vi "Run.vi"(8 "error in (no error)":errorcluster caption="entrée d'erreur (pas d'erreur)", 9 "labels":string[][](array[string]), 10 "X":string[][](array[string]), 11 "Davies_Bouldin_Score.lvclass":refnum<class "Davies_Bouldin_Score.lvclass">) -> (0 "error out":errorcluster caption="sortie d'erreur", 2 "Score":string, 3 "Davies_Bouldin_Score.lvclass":refnum<class "Davies_Bouldin_Score.lvclass">)   [LabVIEW 2020, in "Davies_Bouldin_Score.lvclass"]
doc: "Returns :\n\n- score : float\nThe resulting Davies-Bouldin score."
uses:
  Davies_Bouldin_Score.lvclass
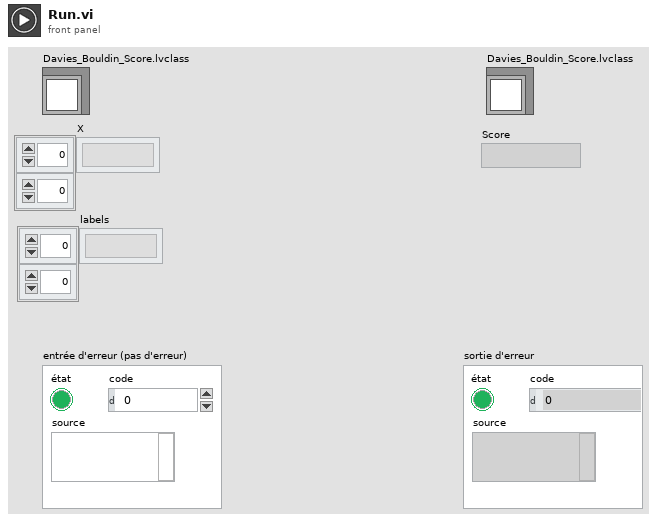
[diagram p1: front panel]
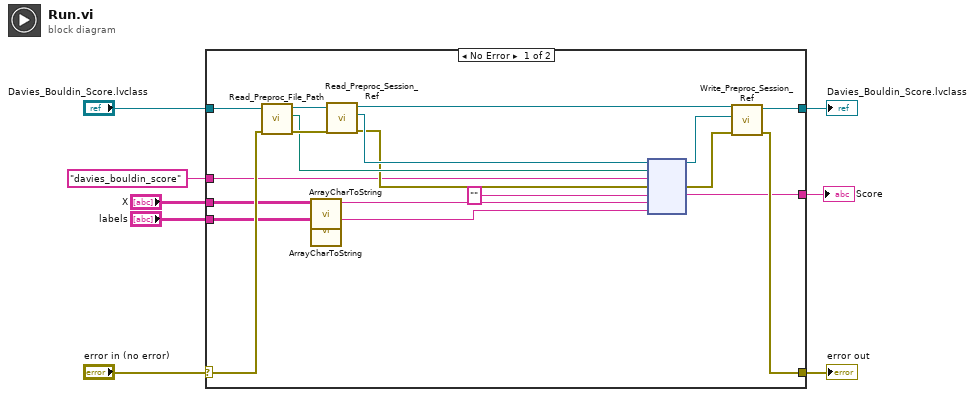
[diagram p0: block diagram]
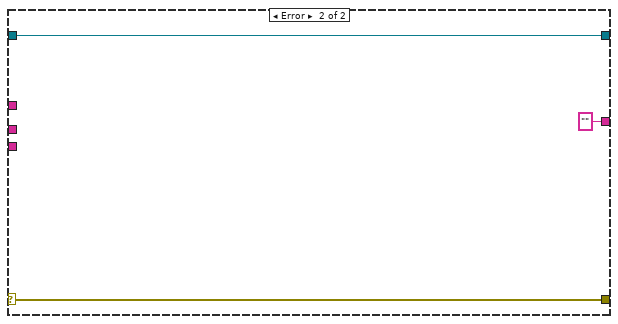
[diagram p2: hidden frame]
diagram:
  n1 = case shown="No Error" "error in (no error)" {
    selector: "error in (no error)" -> [w16 w30]
    tunnel: [w17 w30] -> w7
    tunnel: [w18 w29] -> w5
    tunnel: "Davies_Bouldin_Score.lvclass" -> [w13 w29]
    tunnel: "davies_bouldin_score" -> [w15 _]
    tunnel: [w14 ""] -> w4
    tunnel: "X" -> [w12 _]
    tunnel: "labels" -> [w11 _]
    frame No Error {
      n2 = call-dynamic "Read_Preproc_File_Path.vi"("error in (no error)"=w16, "Python in"=w13) -> ("error out"=w26:errorcluster, "File_Path"=w25:path, "Python out"=w27:refnum<class "Davies_Bouldin_Score.lvclass">)  [unwired: 7 in]
      n3 = call "ArrayCharToString.vi"("TAB"=w12) -> ("Instruction"=w10:string)  [unwired: 10 in]
      n4 = call "ArrayCharToString.vi"("TAB"=w11) -> ("Instruction"=w9:string)  [unwired: 10 in]
      n5 = call-dynamic "Read_Preproc_Session_Ref.vi"("error in (no error)"=w26, "Python in"=w27) -> ("error out"=w23:errorcluster, "Session_ref"=w24:refnum<k35>, "Python out"=w22:refnum<class "Davies_Bouldin_Score.lvclass">)  [unwired: 7 in]
      n6 = node(w24, w25, w15, w23, "", w10, w9) -> (w20:refnum<k35>, w21:errorcluster, w14:string)  [unwired: 2 in, 2 out]
      n7 = call-dynamic "Write_Preproc_Session_Ref.vi"("error in (no error)"=w21, "Session_ref"=w20, "Python in"=w22) -> ("error out"=w17:errorcluster, "Python out"=w18:refnum<class "Davies_Bouldin_Score.lvclass">)  [unwired: 7 in]
    }
    frame Error {
    }
  }
  "error out" <- w7
  "Davies_Bouldin_Score.lvclass" <- w5
  "Score" <- w4
